vi "Circular Buffer (waveform).vi"(6 "History Length [1024]":i32=1024, 7 "reset":bool, 8 "error in":errorcluster, 11 "Waveform in":waveform(dbl)) -> (0 "error out":errorcluster, 3 "Waveform out":waveform(dbl))   [LabVIEW 2019, in "xy_utilities.lvlib"]
doc: "Circular Buffer with controllable reset and history length."
uses:
  xy_utilities.lvlib
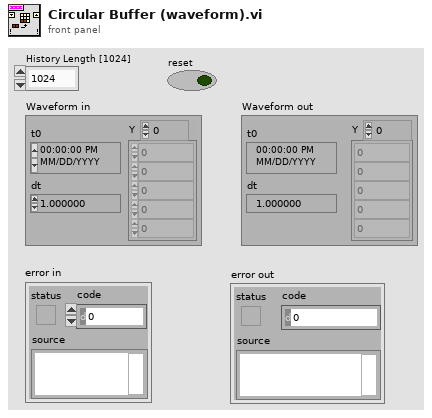
[diagram p1: front panel]
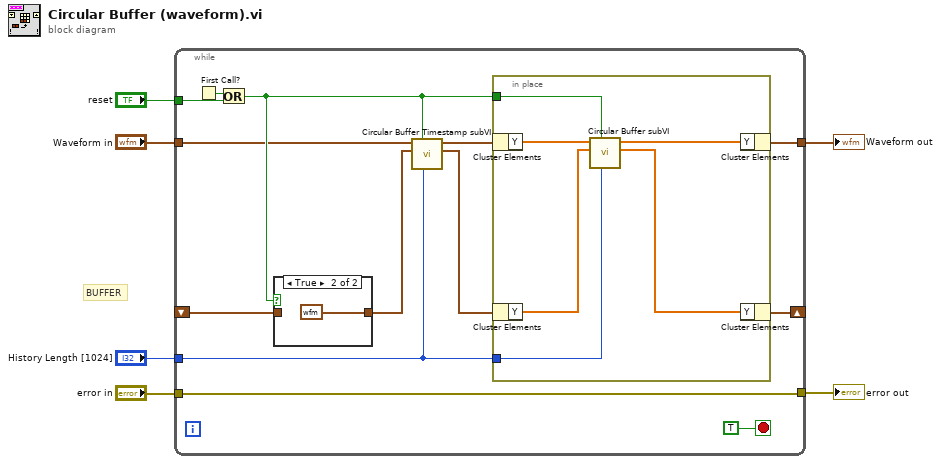
[diagram p0: block diagram]
diagram:
  # "BUFFER"
  n1 = while {
    tunnel: "Waveform in" -> [w10]
    tunnel: [w19] -> w3
    tunnel: "error in" -> [w19]
    tunnel: "reset" -> [w17]
    shift-right: [w13] -> _
    shift-left: _ -> [w15]
    tunnel: "History Length [1024]" -> [w8]
    tunnel: [w14] -> w1
    stop <- TRUE stop-if-true
    n2 = First Call?() -> (First Call?: T/F=w18:bool)
    n3 = Or(x=w18, y=w17) -> (x .or. y?=w11:bool)
    n4 = case shown="True" w11 {
      tunnel: w15 -> [w26 _]
      tunnel: [w26 waveform(dbl) {"t0"=timestamp(0 s since 1904-01-01), "dt"=1.0, "Y"=[]} ("Waveform in")] -> w9
      frame False {
      }
      frame True {
      }
    }
    n5 = call "Circular Buffer Timestamp subVI.vi"("History Length [1024]"=w8, "reset"=w11, "Buffer in"=w9, "Waveform in in"=w10) -> ("Buffer out"=w7:waveform(dbl), "Waveform out"=w12:waveform(dbl))  [unwired: 6 in]
    n6 = in-place {
      in-place-border: w8 -> [w22]
      in-place-border: w11 -> [w24]
      n7 = in-place-cluster #1(w12) -> ("Y"=w21:dbl[])
      n8 = in-place-cluster #2(w7) -> ("Y"=w23:dbl[])
      n9 = call "Circular Buffer subVI.vi"("History Length [1024]"=w22, "Reset"=w24, "Buffer in"=w23, "Array in"=w21) -> ("Buffer out"=w20:dbl[], "Array out"=w25:dbl[])  [unwired: 6 in]
      n10 = in-place-cluster #1("Y"=w25) -> (w14:waveform(dbl))
      n11 = in-place-cluster #2("Y"=w20) -> (w13:waveform(dbl))
    }
  }
  "Waveform out" <- w1
  "error out" <- w3
